vi "AT Finalise Library A.vi"(8 "error in (no error)":errorcluster) -> (0 "error out":errorcluster, 3 "Status":i32)   [LabVIEW 2019]
doc: "Finalise Library\n\nOutput:\n I32 Status\n\nInput:\n void\n\nThis function will free up any resources used by the SDK and should be called whenever the program no longer needs to use any SDK functions. AT_InitialiseLibrary may be called again later by the same process if camera control is again required. Never call FinaliseLibrary if there are camera handles open."
uses:
  atcoreA.dll
  atunpacker.dll
panel:
  out "Cleanup status":i32
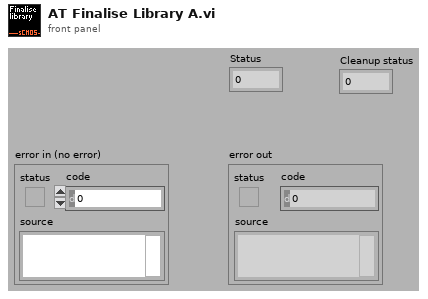
[diagram p1: front panel]
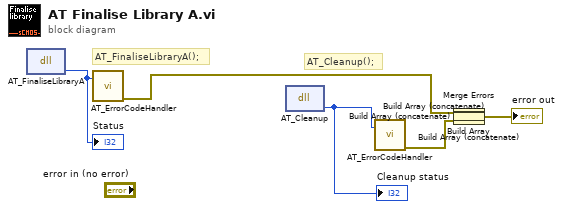
[diagram p0: block diagram]
diagram:
  # "AT_Cleanup();"
  # "AT_FinaliseLibraryA();"
  n1 = dll-call lib="atcoreA.dll" fn="AT_FinaliseLibraryA"() -> ("Status"=w9:i32)  [unwired: 3 in, 2 out]
  "Status" <- w9
  n2 = call "AT_ErrorCodeHandler.vi"("Error"=w9) -> ("error out"=w2:errorcluster)  [unwired: 6 in]
  n3 = dll-call lib="atunpacker.dll" fn="AT_Cleanup"() -> ("return type"=w6:i32)  [unwired: 3 in, 2 out]
  "Cleanup status" <- w6
  n4 = call "AT_ErrorCodeHandler.vi"("Error"=w6) -> ("error out"=w8:errorcluster)  [unwired: 6 in]
  n5 = Build Array(w2, w8) -> (w5:errorcluster[])
  n6 = Build Array (concatenate)(w5) -> (w4:errorcluster[])
  n7 = Build Array (concatenate)(w4) -> (w3:errorcluster[])
  n8 = Build Array (concatenate)(w3) -> (w1:errorcluster[])
  n9 = Merge Errors(w1) -> (→"error out":errorcluster)
